vi "SDT_CreateModTypeString.vi"(11 "mod_type-String":string) -> (2 "mod_type2":u64 format="%016x", 3 "mod_type1":u64 format="%016x")   [LabVIEW 2019]
doc: "This VI is a SubVI to SDT_GenerateMeasureInfoBlock.vi. \nIt formats the ASCII-string describing the module type to two U64 binary integers.to be inserted at the MeasureInfo cluster's parameters 'MeasureInfo_PartB.mod_type1' and 'MeasureInfo_PartB.mod_type2'.\n\ninfo@becker-hickl.com"
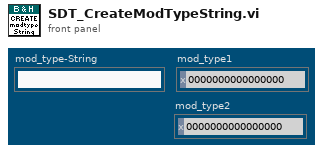
[diagram p1: front panel]
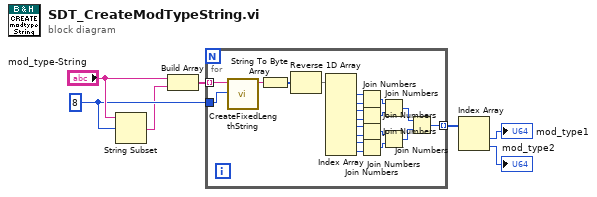
[diagram p0: block diagram]
diagram:
  w5 = 8 ("RequiredStringLength")
  n1 = String Subset(string="mod_type-String", offset (0)=w5) -> (substring=w1:string)  [unwired: 1 in]
  n2 = Build Array("mod_type-String", w1) -> (w2:string[])
  n3 = for {
    tunnel: [w26] -> w7 mode=indexing
    tunnel: w2 -> [w9] mode=indexing
    tunnel: w5 -> [w8]
    n4 = call "CreateFixedLengthString.vi"("RequiredStringLength"=w8, "StringIn"=w9) -> ("DLLString"=w10:string)  [unwired: 8 in, 1 out]
    n5 = String To Byte Array(string=w10) -> (unsigned byte array=w11:u8[])
    n6 = Reverse 1D Array(array=w11) -> (reversed array=w27:u8[])
    n7 = Index Array(array=w27) -> (element #1=w12:u8, element #2=w13:u8, element #3=w14:u8, element #4=w15:u8, element #5=w16:u8, element #6=w17:u8, element #7=w18:u8, element #8=w19:u8)  [unwired: 8 in]
    n8 = Join Numbers(hi=w12, lo=w13) -> ((hi.lo)=w20:u16)
    n9 = Join Numbers(hi=w14, lo=w15) -> ((hi.lo)=w21:u16)
    n10 = Join Numbers(hi=w16, lo=w17) -> ((hi.lo)=w22:u16)
    n11 = Join Numbers(hi=w18, lo=w19) -> ((hi.lo)=w23:u16)
    n12 = Join Numbers(hi=w20, lo=w21) -> ((hi.lo)=w24:u32)
    n13 = Join Numbers(hi=w22, lo=w23) -> ((hi.lo)=w25:u32)
    n14 = Join Numbers(hi=w24, lo=w25) -> ((hi.lo)=w26:u64)
  }
  n15 = Index Array(array=w7) -> (element #1=→"mod_type1":u64, element #2=→"mod_type2":u64)  [unwired: 2 in]
